vi "07Foot_StopDAQ.vi"(0 "task/channels in":refnum<k21>, 11 "error in":errorcluster) -> (4 "task out":refnum<k21>, 15 "error out":errorcluster)   [LabVIEW 2015]
doc: "Stops the task and returns it to the state the task was in before the DAQmx Start Task VI ran or the DAQmx Write VI ran with the <B>autostart</B> input set to TRUE."
uses:
  nilvaiu.dll
panel:
  in  "depth":i32
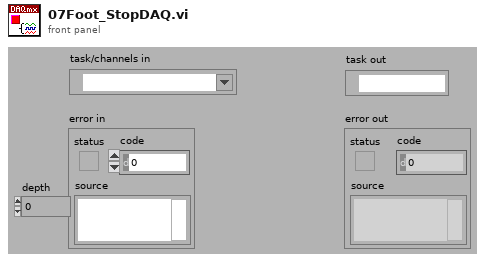
[diagram p1: front panel]
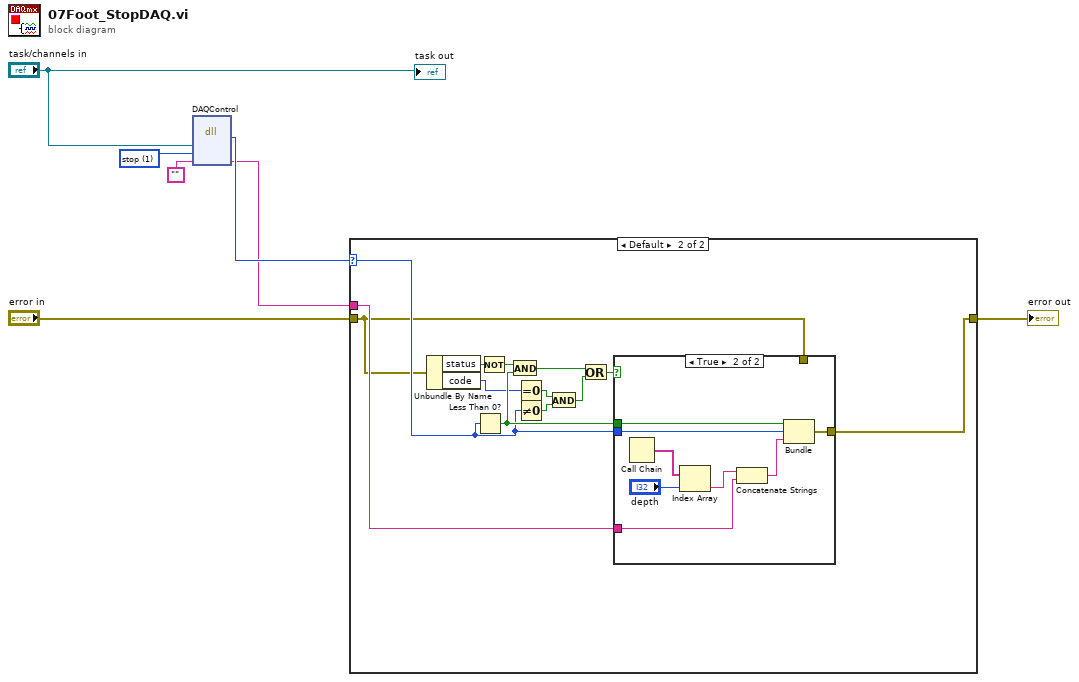
[diagram p0: block diagram]
diagram:
  w5 = u16 1 items=["stop"=1]
  n1 = dll-call lib="nilvaiu.*" fn="DAQControl"("taskID"="task/channels in", "mode"=w5, "extendedErrorInfo"="") -> (w4:i32, "extendedErrorInfo"=w3:string)  [unwired: 3 in, 4 out]
  n2 = case shown="Default" w4 {
    selector: w4 -> [_ w12]
    tunnel: "error in" -> [w8 w9]
    tunnel: [w8 w10] -> w1
    tunnel: w3 -> [_ w11]
    frame 0 {
    }
    frame Default {
      n3 = Unbundle By Name(w9) -> ("status"=w16:bool, "code"=w20:i32)
      n4 = Less Than 0?(x=w12) -> (x < 0?=w21:bool)
      n5 = Not(x=w16) -> (.not. x?=w19:bool)
      n6 = And(x=w19, y=w21) -> (x .and. y?=w17:bool)
      n7 = Equal To 0?(x=w20) -> (x = 0?=w15:bool)
      n8 = Not Equal To 0?(x=w12) -> (x != 0?=w18:bool)
      n9 = And(x=w15, y=w18) -> (x .and. y?=w14:bool)
      n10 = Or(x=w17, y=w14) -> (x .or. y?=w13:bool)
      n11 = case shown="True" w13 {
        tunnel: [w22 w29] -> w10
        tunnel: w12 -> [_ w28]
        tunnel: w21 -> [_ w27]
        tunnel: w9 -> [w22 _]
        tunnel: w11 -> [_ w23]
        frame False {
        }
        frame True {
          n12 = Call Chain() -> (call chain=w26:string[])
          n13 = Index Array(array=w26, index="depth") -> (element=w24:string)
          n14 = Concatenate Strings(w24, w23) -> (w30:string)
          n15 = Bundle(w27, w28, w30) -> (w29:errorcluster)  [unwired: 1 out]
        }
      }
    }
  }
  "error out" <- w1
  "task out" <- "task/channels in"
